vi "HMI Main.vi"() -> ()   [LabVIEW 2011]
uses:
  <vilib>/dex/Flush And Wait Empty Condition.ctl
panel:
  in  "Recipe":T1(array[cluster])=[{"Temp Setpoint"=26.0, "pH Setpoint"=1.7, "Agitation ON"=TRUE, "Intake ON"=FALSE, "Waste ON"=TRUE, "Time (s)"=5.0}, {"Temp Setpoint"=30.0, "pH Setpoint"=1.3, "Agitation ON"=FALSE, "Intake ON"=TRUE, "Waste ON"=FALSE, "Time (s)"=5.0}, {"Temp Setpoint"=27.0, "pH Setpoint"=1.5, "Agitation ON"=TRUE, "Intake ON"=FALSE, "Waste ON"=TRUE, "Time (s)"=5.0}]
  in  "error in":errorcluster
  out "Waste ON":bool
  out "Intake ON":bool
  out "Agitation ON":bool
  in  "Abort Recipe":bool
  out "error out":errorcluster
  in  "Target IP Address":string="10.0.60.140"
  in  "Exit":bool
  in  "Run":bool
  in  "pH Override":bool
  in  "Temp Override":bool
  out "pH":dbl
  in  "pH Setpoint":dbl
  out "Temp":dbl
  in  "Temp Setpoint":dbl
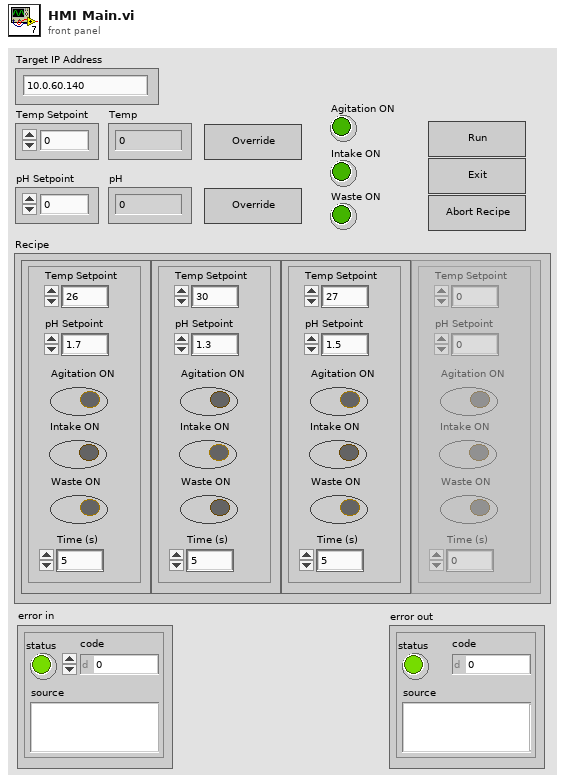
[diagram p1: front panel]
types:
  T1 = cluster{"Temp Setpoint":dbl, "pH Setpoint":dbl, "Agitation ON":bool, "Intake ON":bool, "Waste ON":bool, "Time (s)":dbl}[]
  T2 = typedef "Flush And Wait Empty Condition.ctl" = u8
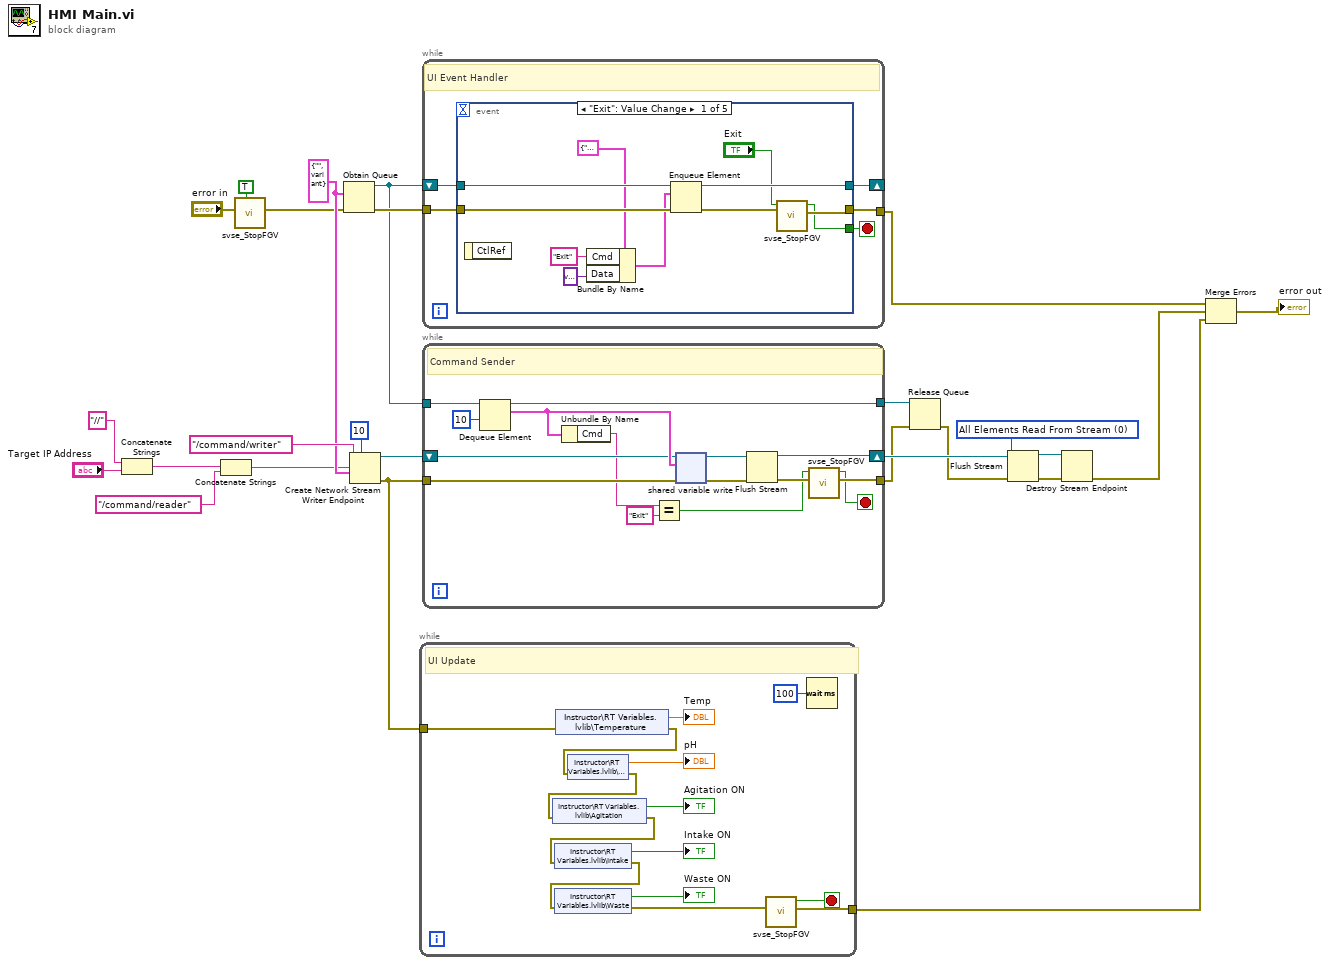
[diagram p0: block diagram]
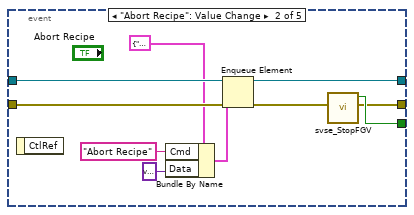
[diagram p2: hidden frame]
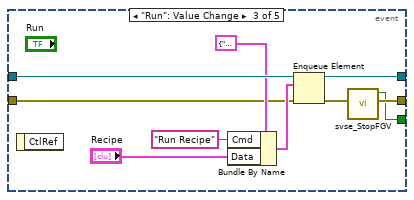
[diagram p3: hidden frame]
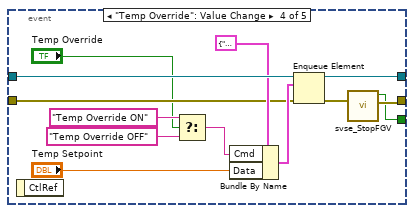
[diagram p4: hidden frame]
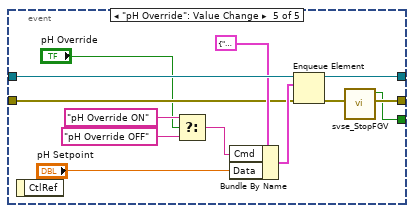
[diagram p5: hidden frame]
diagram:
  w8 = T2 0 items=["All Elements Read From Stream", "All Elements Available for Reading"] ("wait condition")
  w22 = cluster{"Cmd":string, "Data":variant} {"Cmd"="", "Data"=variant}
  n1 = Concatenate Strings("//" ("reader url"), "Target IP Address") -> (w19:string)
  n2 = Concatenate Strings(w19, "/command/reader" ("reader url")) -> (w17:string)
  n3 = call "svse_StopFGV.vi"("Reset (F)"=TRUE, "error in"="error in") -> ("error out"=w11:errorcluster)  [unwired: 8 in, 1 out]
  n4 = Obtain Queue(element data type=w22, error in (no error)=w11) -> (queue out=w25:refnum<queue>, error out=w26:errorcluster)  [unwired: 3 in, 1 out]
  n5 = Create Network Stream Writer Endpoint(7:10 ("writer buffer size"), 9:w22, 10:w17, 11:"/command/writer" ("writer name")) -> (0:w14:errorcluster, 3:w23:refnum<k21>)  [unwired: 2 in]
  n6 = while {
    tunnel: w14 -> [w31]
    tunnel: [w33] -> w13
    stop <- w34 stop-if-true
    # "UI Update"
    n7 = shared-variable "Instructor\\RT Variables.lvlib\\Temperature"(error in=w31) -> (→"Temp":dbl, error out=w30:errorcluster)
    n8 = shared-variable "Instructor\\RT Variables.lvlib\\pH"(error in=w30) -> (→"pH":dbl, error out=w29:errorcluster)
    n9 = shared-variable "Instructor\\RT Variables.lvlib\\Agitation"(error in=w29) -> (→"Agitation ON":bool, error out=w28:errorcluster)
    n10 = shared-variable "Instructor\\RT Variables.lvlib\\Intake"(error in=w28) -> (→"Intake ON":bool, error out=w27:errorcluster)
    n11 = shared-variable "Instructor\\RT Variables.lvlib\\Waste"(error in=w27) -> (→"Waste ON":bool, error out=w35:errorcluster)
    n12 = call "svse_StopFGV.vi"("error in"=w35) -> ("error out"=w33:errorcluster, "Stop?"=w34:bool)  [unwired: 9 in]
    n13 = Wait (ms)(milliseconds to wait=u32 100) -> ()  [unwired: 1 out]
  }
  n14 = while {
    shift-right: [w41] -> _
    shift-left: w25 -> [w44]
    tunnel: w26 -> [w43]
    tunnel: [w42] -> w1
    stop <- w45 stop-if-true
    # "UI Event Handler"
    n15 = event shown="[0] \"Exit\": Value Change" {
      selector: _ -> [_ _ _ _ _]
      dyn-events: _ -> [_ _ _ _ _]
      timeout: _ -> [_ _ _ _ _]
      tunnel: [w46 w58 w68 w77 w90] -> w45
      tunnel: w44 -> [w56 w66 w76 w89 w102]
      tunnel: w43 -> [w54 w64 w71 w84 w98]
      tunnel: [w49 w57 w69 w78 w91] -> w42
      tunnel: [w55 w65 w72 w86 w99] -> w41
      event "Exit": Value Change {
        n16 = event-data() -> ()  [unwired: 1 in, 1 out]
        n17 = Bundle By Name(cluster=cluster{"Cmd":string, "Data":variant} {"Cmd"="", "Data"=variant}, "Cmd"="Exit", "Data"=variant) -> (w51:cluster{"Cmd":string, "Data":variant})
        n18 = Enqueue Element(queue=w56, element=w51, error in (no error)=w54) -> (queue out=w55:refnum<queue>, error out=w48:errorcluster)  [unwired: 1 in, 1 out]
        n19 = call "svse_StopFGV.vi"("error in"=w48, "User stop? (F)"="Exit") -> ("error out"=w49:errorcluster, "Stop?"=w46:bool)  [unwired: 8 in]
      }
      event "Abort Recipe": Value Change {
        n20 = event-data() -> ()  [unwired: 1 in, 1 out]
        n21 = Bundle By Name(cluster=cluster{"Cmd":string, "Data":variant} {"Cmd"="", "Data"=variant}, "Cmd"="Abort Recipe", "Data"=variant) -> (w61:cluster{"Cmd":string, "Data":variant})
        n22 = Enqueue Element(queue=w66, element=w61, error in (no error)=w64) -> (queue out=w65:refnum<queue>, error out=w59:errorcluster)  [unwired: 1 in, 1 out]
        n23 = call "svse_StopFGV.vi"("error in"=w59) -> ("error out"=w57:errorcluster, "Stop?"=w58:bool)  [unwired: 9 in]
      }
      event "Run": Value Change {
        n24 = event-data() -> ()  [unwired: 1 in, 1 out]
        n25 = Bundle By Name(cluster=cluster{"Cmd":string, "Data":variant} {"Cmd"="", "Data"=variant}, "Cmd"="Run Recipe", "Data"="Recipe") -> (w74:cluster{"Cmd":string, "Data":variant})
        n26 = Enqueue Element(queue=w76, element=w74, error in (no error)=w71) -> (queue out=w72:refnum<queue>, error out=w70:errorcluster)  [unwired: 1 in, 1 out]
        n27 = call "svse_StopFGV.vi"("error in"=w70) -> ("error out"=w69:errorcluster, "Stop?"=w68:bool)  [unwired: 9 in]
      }
      event "Temp Override": Value Change {
        n28 = event-data() -> ()  [unwired: 1 in, 1 out]
        n29 = Select(t="Temp Override ON" ("Cmd"), s="Temp Override", f="Temp Override OFF" ("Cmd")) -> (s? t:f=w80:string)
        n30 = Bundle By Name(cluster=cluster{"Cmd":string, "Data":variant} {"Cmd"="", "Data"=variant}, "Cmd"=w80, "Data"="Temp Setpoint") -> (w87:cluster{"Cmd":string, "Data":variant})
        n31 = Enqueue Element(queue=w89, element=w87, error in (no error)=w84) -> (queue out=w86:refnum<queue>, error out=w79:errorcluster)  [unwired: 1 in, 1 out]
        n32 = call "svse_StopFGV.vi"("error in"=w79) -> ("error out"=w78:errorcluster, "Stop?"=w77:bool)  [unwired: 9 in]
      }
      event "pH Override": Value Change {
        n33 = event-data() -> ()  [unwired: 1 in, 1 out]
        n34 = Select(t="pH Override ON" ("Cmd"), s="pH Override", f="pH Override OFF" ("Cmd")) -> (s? t:f=w95:string)
        n35 = Bundle By Name(cluster=cluster{"Cmd":string, "Data":variant} {"Cmd"="", "Data"=variant}, "Cmd"=w95, "Data"="pH Setpoint") -> (w100:cluster{"Cmd":string, "Data":variant})
        n36 = Enqueue Element(queue=w102, element=w100, error in (no error)=w98) -> (queue out=w99:refnum<queue>, error out=w92:errorcluster)  [unwired: 1 in, 1 out]
        n37 = call "svse_StopFGV.vi"("error in"=w92) -> ("error out"=w91:errorcluster, "Stop?"=w90:bool)  [unwired: 9 in]
      }
    }
  }
  n38 = while {
    tunnel: w25 -> [w117]
    shift-right: [w109] -> w9
    shift-left: w23 -> [w114]
    tunnel: w14 -> [w112]
    tunnel: [w106] -> w3
    tunnel: [w104] -> w4
    stop <- w105 stop-if-true
    # "Command Sender"
    n39 = Dequeue Element(queue=w117, timeout in ms (-1)=10) -> (queue out=w104:refnum<queue>, element=w115:cluster{"Cmd":string, "Data":variant})  [unwired: 1 in, 2 out]
    n40 = Unbundle By Name(w115) -> ("Cmd"=w111:string)
    n41 = Equal?(x=w111, y="Exit") -> (x = y?=w103:bool)
    n42 = shared-variable-write ("Write Single Element to Stream")(w114, w112, w115) -> (w110:refnum<k21>, w108:errorcluster)  [unwired: 1 in, 1 out]
    n43 = Flush Stream(8:w108, 11:w110) -> (0:w107:errorcluster, 3:w109:refnum<k21>)  [unwired: 2 in, 1 out]
    n44 = call "svse_StopFGV.vi"("error in"=w107, "User stop? (F)"=w103) -> ("error out"=w106:errorcluster, "Stop?"=w105:bool)  [unwired: 8 in]
  }
  n45 = Release Queue(queue=w4, error in (no error)=w3) -> (error out=w2:errorcluster)  [unwired: 1 in, 2 out]
  n46 = Flush Stream(8:w2, 10:w8, 11:w9) -> (0:w6:errorcluster, 3:w7:refnum<k21>)  [unwired: 1 in, 1 out]
  n47 = Destroy Stream Endpoint(8:w6, 11:w7) -> (0:w5:errorcluster)
  n48 = Merge Errors(w1, w5, w13) -> (→"error out":errorcluster)
